vi "RobotMain.vi"() -> ()   [LabVIEW 2018]
panel:
  out "Input 2":dbl(knob) scale=0.0..10.0
  out "Input 1":dbl(knob) scale=0.0..10.0
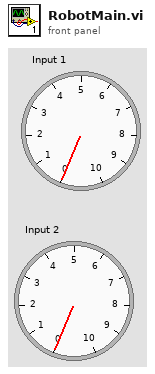
[diagram p1: front panel]
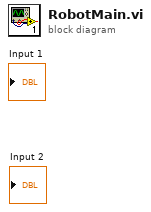
[diagram p0: block diagram]
diagram:
